vi "meth.RecurseReturn.vi"(7 "class.GLue in":refnum<class "class.GLue.lvclass">) -> (8 "class.GLue out":refnum<class "class.GLue.lvclass">)   [LabVIEW 2014, in "GLue.lvlib" / "class.GLue.lvclass"]
uses:
  class.GLue.lvclass
  class.GLue.lvclass/class.GLue.ctl
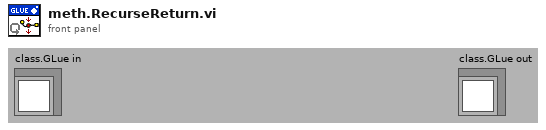
[diagram p1: front panel]
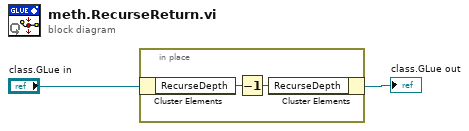
[diagram p0: block diagram]
diagram:
  n1 = in-place {
    n2 = in-place-cluster #1("class.GLue in") -> ("RecurseDepth"=w4:i32)
    n3 = Decrement(x=w4) -> (x-1=w3:i32)
    n4 = in-place-cluster #1("RecurseDepth"=w3) -> (→"class.GLue out":refnum<class "class.GLue.lvclass">)
  }
